vi "FIFO Bucket.vi"() -> ()   [LabVIEW 2012]
doc: "This VI demonstrates how elements are written to and read from a Target-Scoped FIFO on FPGA. When the user selects write, elements will be written to the FIFO in increasing order. If the FIFO runs out of room to write the data, the FIFO Full LED will become true. When the user selects to read from the FIFO, a different loop will begin to read from the FIFO one element at a time and the element will be displayed in the Element Read indicator. If the FIFO runs out of elements to read, the FIFO Empty LED will become true. The bucket is used to keep track of how many elements are currently in the FIFO. This number is calculated by taking the number of successful writes to the FIFO and subtracting the number of successful reads."
uses:
  <vilib>/rvi/Emulation/niFpgaSctlEmulationGetInTimedLoop.vi
  <vilib>/rvi/Emulation/niFpgaSctlEmulationGlobalWrite.vi
  <vilib>/rvi/DataTransferAndStorage/Container/Common/niFpgaContainerGetUniqueNameForEmu.vi
  <vilib>/rvi/FIFO/Fifo_Resource/nirvififoEmulationSetSize.vi
  <vilib>/rvi/Emulation/niFpgaSctlEmulationFifoFullMgr.vi
  <vilib>/rvi/errors/niFpgaSetErrorForExecOnDevCompSimple.vi
  <vilib>/rvi/eio/common/nirviEmuReportErrorAndStop.vi
  <vilib>/rvi/Emulation/niFpgaSctlEmulationResourceMgr.vi
  <vilib>/rvi/DataTransferAndStorage/Container/XNode/niFpgaContainer.xnode
  <vilib>/rvi/FIFO/Fifo_Resource/nirvififoEmulationRead.vi
  <vilib>/rvi/FIFO/Fifo_Resource/nirvififoEmulationGetNumberOfElementsToRead.vi
  <vilib>/rvi/FIFO/Fifo_Resource/nirvififoEmulationWrite.vi
panel:
  out "Element Read":u16
  out "FIFO Underflow":bool
  out "FIFO Overflow":bool
  out "Bucket":u16(slide) scale=0.0..36.0
  in  "Read":bool
  in  "Write":bool
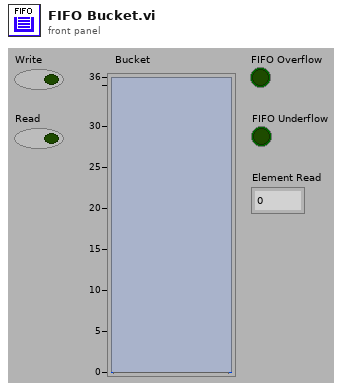
[diagram p1: front panel]
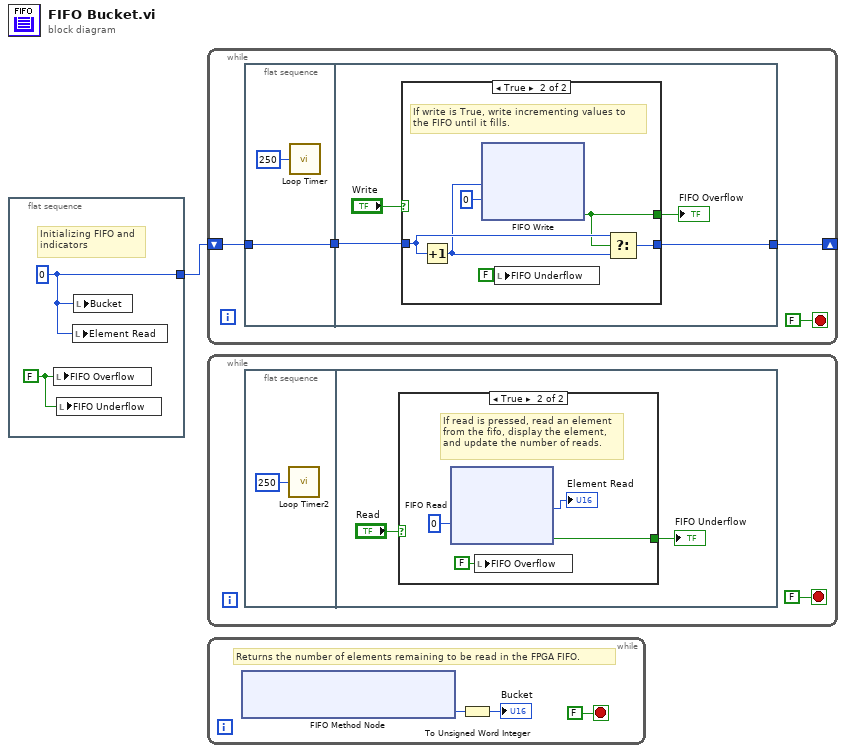
[diagram p0: block diagram]
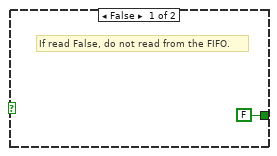
[diagram p2: hidden frame]
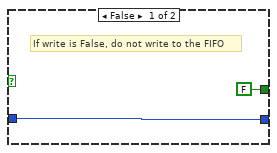
[diagram p3: hidden frame]
diagram:
  n1 = flat-sequence {
    tunnel: [w3] -> w1
    frame #0 {
      w2 = FALSE ("FIFO Full")
      w3 = u16 0 ("writes")
      # "Initializing FIFO and\nindicators"
      n2 = local write "FIFO Overflow"(w2) -> ()
      n3 = local write "FIFO Underflow"(w2) -> ()
      n4 = local write "Element Read"(w3) -> ()
      n5 = local write "Bucket"(w3) -> ()
    }
  }
  n6 = while {
    shift-right: [w4] -> _
    shift-left: w1 -> [w5]
    stop <- FALSE stop-if-true
    n7 = flat-sequence {
      tunnel: [w9] -> w6
      tunnel: w5 -> [w9]
      tunnel: w6 -> [w12]
      tunnel: [w11] -> w4
      frame #0 {
        n8 = call "Loop Timer"("Count(mSec)"=u32 250) -> ()  [unwired: 1 out]
      }
      frame #1 {
        n9 = case shown="True" "Write" {
          tunnel: w12 -> [w15 w20]
          tunnel: [w15 w21] -> w11
          tunnel: [FALSE ("Timed Out?") w16] -> w10
          frame False {
            # "If write is False, do not write to the FIFO"
          }
          frame True {
            # "If write is True, write incrementing values to the FIFO until it fills."
            n10 = Increment(x=w20) -> (x+1=w19:u16)
            n11 = xnode ("FIFO Write")("Element"=w19, "Timeout"=0) -> ("Timed Out?"=w16:bool)  [unwired: 1 in, 1 out]
            n12 = local write "FIFO Underflow"(FALSE ("FIFO Full")) -> ()
            n13 = Select(t=w20, s=w16, f=w19) -> (s? t:f=w21:u16)
          }
        }
        "FIFO Overflow" <- w10
      }
    }
  }
  n14 = while {
    stop <- FALSE stop-if-true
    n15 = flat-sequence {
      frame #0 {
        n16 = call "Loop Timer2"("Count(mSec)"=u32 250) -> ()  [unwired: 1 out]
      }
      frame #1 {
        n17 = case shown="True" "Read" {
          tunnel: [FALSE ("Timed Out?") w27] -> w24
          frame False {
            # "If read False, do not read from the FIFO."
          }
          frame True {
            # "If read is pressed, read an element\nfrom the fifo, display the element,\nand update the number of reads."
            n18 = xnode ("FIFO Read")("Timeout"=0) -> ("Element"=→"Element Read":u16, "Timed Out?"=w27:bool)  [unwired: 1 in, 1 out]
            n19 = local write "FIFO Overflow"(FALSE ("FIFO Full")) -> ()
          }
        }
        "FIFO Underflow" <- w24
      }
    }
  }
  n20 = while {
    stop <- FALSE stop-if-true
    # "Returns the number of elements remaining to be read in the FPGA FIFO."
    n21 = xnode ("FIFO Method Node")() -> ("Number of Elements to Read"=w32:u32)  [unwired: 1 in, 1 out]
    n22 = To Unsigned Word Integer(number=w32) -> (unsigned 16bit integer=→"Bucket":u16)
  }
